vi "CRYReplace Statistics Curve Name.vi"(6 "IsMessage":bool, 8 "Hardware Setup In":string, 9 "Step Set up In":string, 10 "Setup in":T1={"No.VI"=0, "Category"="", "StepName"="", "Seq setup flattened"="", "Comment"="", "Steps config."=[], "Jump config"=[], "Start"=0.0, "Increment"=0.0, "Name"="Pa", "Unit"="Pa", "Y data"=1, "Y prefix"="", "Y dB ref"=1.0, "Y unit"="", "Repeat State Array"=[]} {"Repeat State Array"."Start" format="%#_5g"; "Y dB ref" format="%.1f"; "Y data" items=["dB", "Lin"]; "Start" format="%#_5g"}, 11 "Type In":string) -> (0 "RunFlag":bool, 3 "Inserted Names Out":string[](array[string]))   [LabVIEW 2013]
uses:
  Typedef Control/CRYStep.ctl
  Typedef Control/CRYData Cluster Array.ctl
  Typedef Control/CRYData Cluster.ctl
  CRYMainGlobal.vi
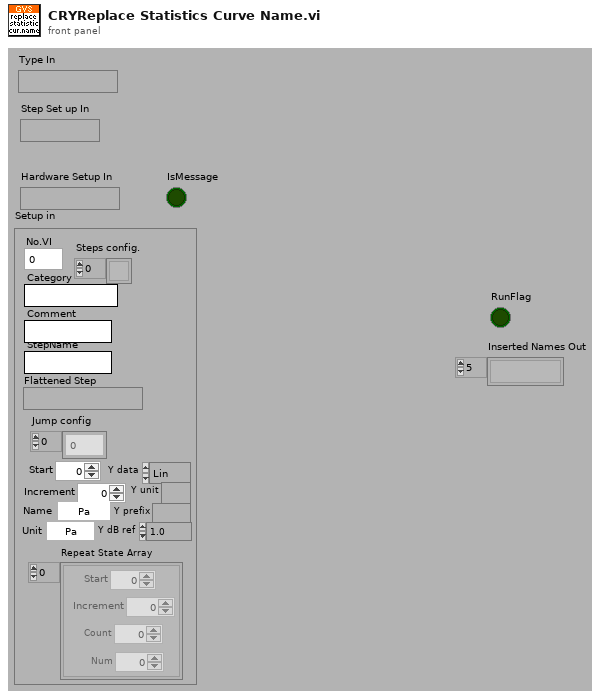
[diagram p1: front panel]
types:
  T1 = typedef "CRYStep.ctl" = cluster{"No.VI":i32, "Category":string, "StepName":string, "Seq setup flattened":string, "Comment":string, "Steps config.":bool[], "Jump config":i32[], "Start":dbl, "Increment":dbl, "Name":string, "Unit":string, "Y data":u16, "Y prefix":string, "Y dB ref":dbl, "Y unit":string, "Repeat State Array":cluster{"Start":dbl, "Increment":dbl, "Count":i32, "Num":i32}[]}
  T2 = typedef "CRYData Cluster Array.ctl" = T3[]
  T3 = typedef "CRYData Cluster.ctl" = cluster{"Name":string, "Curve":cluster{"x":dbl, "y":dbl, "z":dbl}[], "X data":u16, "Y data":u16, "Z data":u16, "X axis":u16, "Y axis":u16, "Z axis":u16, "X unit":string, "Y unit":string, "Z unit":string, "X dB ref":dbl, "Y dB ref":dbl, "Z dB ref":dbl, "single val":bool, "protected":bool, "display X":bool, "display Y":bool, "display Z":bool, "Test Info":string, "Step No.":i32, "Plot Settings":cluster{"Color":u32, "Interpolation":u8, "Point Style":u8, "Line Style":u8, "Point Color":u32, "Line Width":u8, "Bar Plot Style":u8, "Fill To":i16}, "AutoProtect":bool}
  T4 = cluster{"Start":dbl, "Increment":dbl, "Count":i32, "Num":i32}[]
  T5 = typedef "CRYStatistic cluster.ctl" = cluster{"Mode":u16, "No.Ranked(BF)":i32, "No.Ranked(WF)":i32, "Absolute Margin Standard Deviation":bool, "+/- sigma Res":i32, "Margin Standard Deviation":bool, "Margin Mean":bool, "Overall Yield":bool, "Individual Limits Yield":bool, "LSL Unit":string, "USL Unit\n":string, "LSL":dbl, "USL":dbl, "Worst Fit to Average":bool, "Best Fit to Average":bool, "Ppk":bool, "Pp":bool, "Absolute Standard Deviation":bool, "+/- sigma Dat":i32, "Standard Deviation ":bool, "Mean":bool, "Min ":bool, "Max ":bool, "No.of Curves Selected":i32, "Curves":string[], " Results":string[], "Name":string, "Help":string, "Tab Value":enum32{"Setting", "Help"}, "Work in":u16, "Mode xyz":u16}
  T6 = cluster{"Max ":bool, "Min ":bool, "Mean":bool, "Absolute Standard Deviation":bool, "Standard Deviation ":bool, "Pp":bool, "Ppk":bool, "Best Fit to Average":bool, "Worst Fit to Average":bool}
  T7 = cluster{"Individual Limits Yield":bool, "Overall Yield":bool, "Margin Mean":bool, "Absolute Margin Standard Deviation":bool, "Margin Standard Deviation":bool}
  T8 = typedef "CRYResult Cluster.ctl" = cluster{"Name":string, "Margin":dbl, "unit":string, "Verdict":bool, "Limit":string, "Max/Min":string, "protected":bool, "Step No.":i32, "Test Info":string, "AutoProtect":bool}
  T9 = enum32{"English", "Chinese", "Korean", "Japanese", "Russian", "Chinese traditional"}
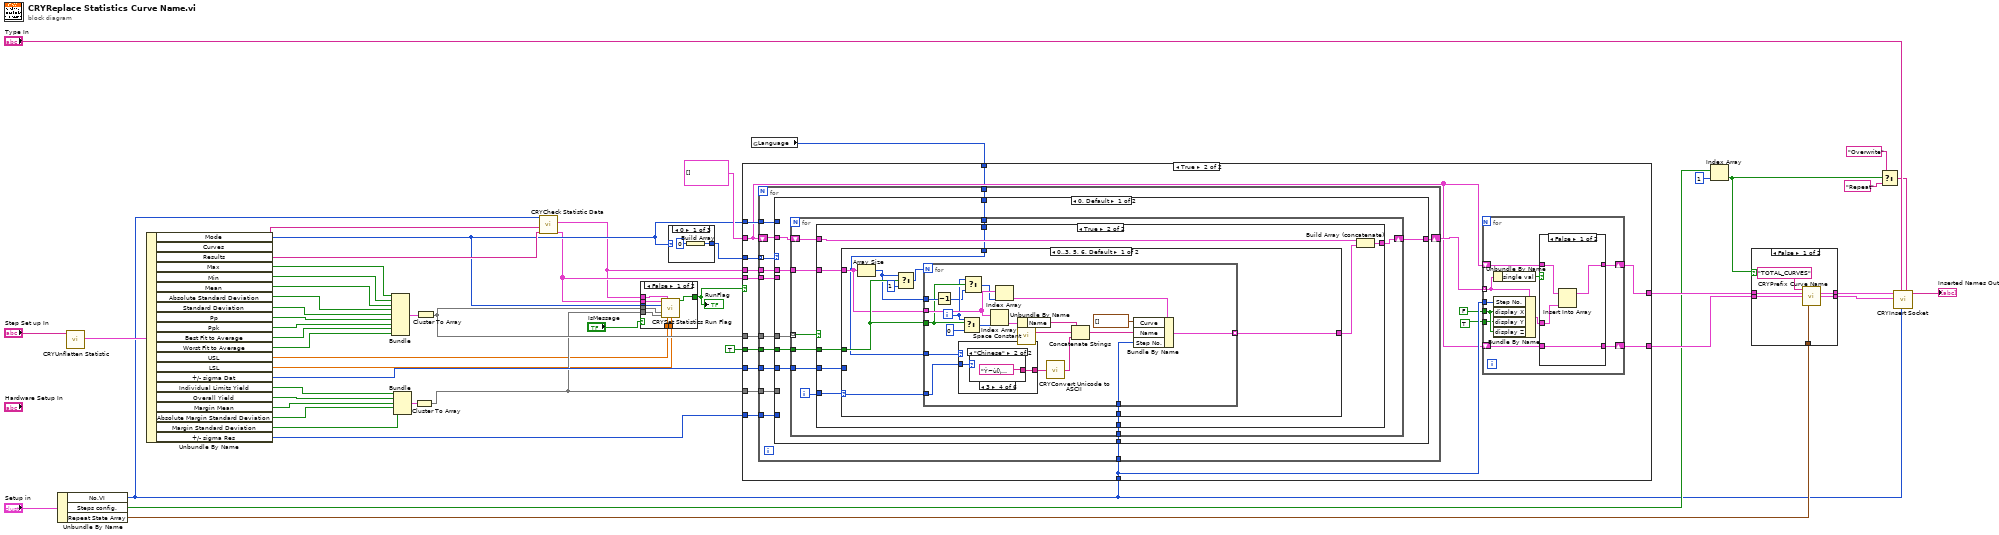
[diagram p0: block diagram]
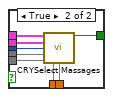
[diagram p2: hidden frame]
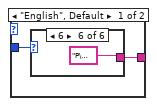
[diagram p6: hidden frame]
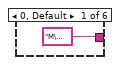
[diagram p7: hidden frame]
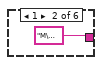
[diagram p8: hidden frame]
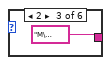
[diagram p9: hidden frame]
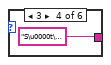
[diagram p10: hidden frame]
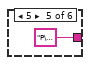
[diagram p11: hidden frame]
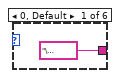
[diagram p12: hidden frame]
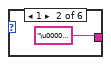
[diagram p13: hidden frame]
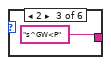
[diagram p14: hidden frame]
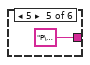
[diagram p15: hidden frame]
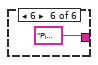
[diagram p16: hidden frame]
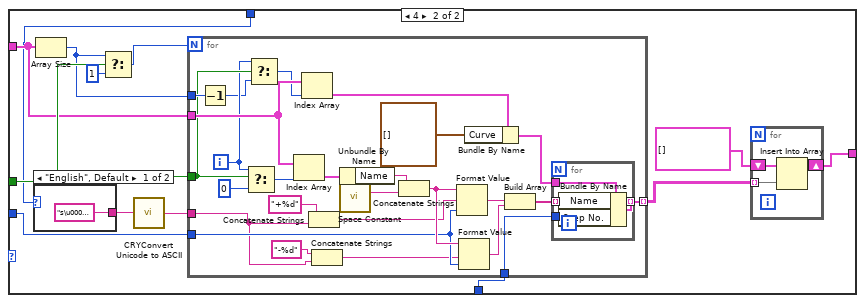
[diagram p17: hidden frame]
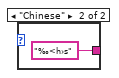
[diagram p18: hidden frame]
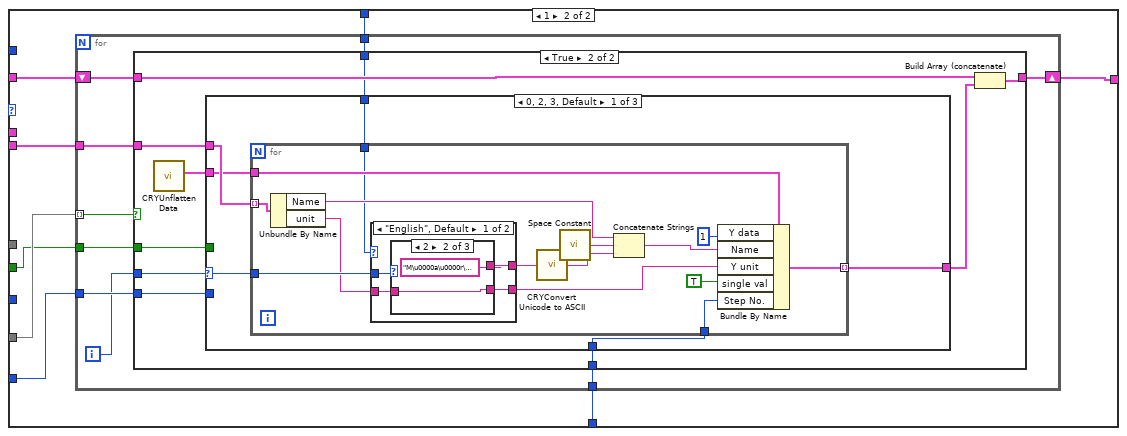
[diagram p19: hidden frame]
diagram:
  n1 = Unbundle By Name("Setup in") -> ("No.VI"=w10:i32, "Steps config."=w16:bool[], "Repeat State Array"=w15:T4)
  n2 = call "CRYUnflatten Statistic.vi"("Flatten Statistics"="Step Set up In") -> ("Statistics"=w29:T5)  [unwired: 10 out]
  n3 = Unbundle By Name(w29) -> ("Mode"=w9:u16, "Curves"=w12:string[], "Results"=w11:string[], "Max"=w47:bool, "Min"=w46:bool, "Mean"=w45:bool, "Absolute Standard Deviation"=w44:bool, "Standard Deviation"=w43:bool, "Pp"=w42:bool, "Ppk"=w41:bool, "Best Fit to Average"=w40:bool, "Worst Fit to Average"=w39:bool, "USL"=w6:dbl, "LSL"=w5:dbl, "+/- sigma Dat"=w32:i32, "Individual Limits Yield"=w37:bool, "Overall Yield"=w36:bool, "Margin Mean"=w35:bool, "Absolute Margin Standard Deviation"=w34:bool, "Margin Standard Deviation"=w33:bool, "+/- sigma Res"=w31:i32)
  n4 = Bundle("Max"=w47, "Min"=w46, "Mean"=w45, "Absolute Standard Deviation"=w44, "Standard Deviation"=w43, "Pp"=w42, "Ppk"=w41, "Best Fit to Average"=w40, "Worst Fit to Average"=w39) -> (w48:T6)  [unwired: 1 out]
  n5 = Bundle("Individual Limits Yield"=w37, "Overall Yield"=w36, "Margin Mean"=w35, "Absolute Margin Standard Deviation"=w34, "Margin Standard Deviation"=w33) -> (w38:T7)  [unwired: 1 out]
  n6 = Cluster To Array(cluster=w38) -> (array=w7:bool[])
  n7 = Cluster To Array(cluster=w48) -> (array=w8:bool[])
  n8 = call "CRYCheck Statistic Data.vi"("Results"=w11, "Curves"=w12, "No.VI"=w10) -> ("Result Out"=w4:T8[], "Data Out"=w3:T2)  [unwired: 7 in]
  n9 = case shown="False" "IsMessage" {
    tunnel: w9 -> [w56 w66]
    tunnel: w8 -> [w55 w65]
    tunnel: w7 -> [w54 w64]
    tunnel: w6 -> [w53 w63]
    tunnel: w5 -> [w52 w62]
    tunnel: w4 -> [w57 w61]
    tunnel: w3 -> [w58 w60]
    tunnel: [w51 w59] -> w2
    frame False {
      n10 = call "CRYSet Statistics Run Flag.vi"("Results in"=w57, "Data in"=w58, "Mode"=w56, "Dat_State"=w55, "Res_state"=w54, "USL"=w53, "LSL"=w52) -> ("Run flag"=w51:bool)  [unwired: 7 in, 1 out]
    }
    frame True {
      n11 = call "CRYSelect Massages.vi"("Data in"=w60, "Results in"=w61, "Mode"=w66, "Dat_State"=w65, "Res_state"=w64, "USL"=w63, "LSL"=w62) -> ("Run flag"=w59:bool)  [unwired: 3 in, 5 out]
    }
  }
  "RunFlag" <- w2
  n12 = case shown="0" w9 {
    tunnel: [w67 w69 w71] -> w30
    frame 0 {
      n13 = Build Array(0 ("No.Ranked(WF)")) -> (w67:i32[])
    }
    frame 1 {
      n14 = Build Array(1 ("No.Ranked(WF)")) -> (w69:i32[])
    }
    frame 2, Default {
      n15 = Build Array(0 ("No.Ranked(WF)"), 1 ("No.Ranked(WF)")) -> (w71:i32[])
    }
  }
  n16 = global read "CRYMainGlobal.vi" "Language"() -> (w13:T9)
  n17 = case shown="True" w2 {
    tunnel: w32 -> [_ w91]
    tunnel: w31 -> [_ w90]
    tunnel: w30 -> [_ w89]
    tunnel: w8 -> [_ w88]
    tunnel: w7 -> [_ w87]
    tunnel: w9 -> [_ w86]
    tunnel: TRUE ("On/Off Line") -> [_ w85]
    tunnel: w3 -> [_ w84]
    tunnel: w4 -> [_ w83]
    tunnel: [w74 w81] -> w22
    tunnel: [w74 w80] -> w21
    tunnel: w10 -> [_ w79]
    tunnel: T2 [] ("Data in") -> [w74 w78]
    tunnel: w13 -> [_ w77]
    frame False {
    }
    frame True {
      n18 = for {
        tunnel: w89 -> [w104] mode=indexing
        tunnel: w88 -> [w103]
        tunnel: w87 -> [w102]
        tunnel: w91 -> [w101]
        tunnel: w90 -> [w100]
        tunnel: w84 -> [w99]
        tunnel: w86 -> [w97]
        shift-right: [w96] -> w82
        shift-left: w78 -> [w98]
        tunnel: w85 -> [w95]
        tunnel: w83 -> [w94]
        tunnel: w79 -> [w93]
        tunnel: w77 -> [w92]
        n19 = case shown="0, Default" w104 {
          tunnel: w103 -> [w112 _]
          tunnel: w102 -> [_ w231]
          tunnel: w101 -> [w111 _]
          tunnel: w100 -> [_ w232]
          tunnel: w99 -> [w110 _]
          tunnel: w98 -> [w109 w230]
          tunnel: w97 -> [_ _]
          tunnel: [w108 w229] -> w96
          tunnel: w95 -> [w107 w227]
          tunnel: w94 -> [_ w228]
          tunnel: w93 -> [w106 w226]
          tunnel: w92 -> [w105 w225]
          frame 0, Default {
            n20 = for {
              tunnel: w112 -> [w120] mode=indexing
              tunnel: w111 -> [w121]
              tunnel: w110 -> [w118]
              shift-right: [w116] -> w108
              shift-left: w109 -> [w117]
              tunnel: w107 -> [w115]
              tunnel: w106 -> [w114]
              tunnel: w105 -> [w113]
              i -> [w119]
              n21 = case shown="True" w120 {
                tunnel: w119 -> [_ w129]
                tunnel: w121 -> [_ w125]
                tunnel: w118 -> [_ w128]
                tunnel: w117 -> [w122 w131]
                tunnel: [w122 w130] -> w116
                tunnel: w115 -> [_ w127]
                tunnel: w114 -> [_ w124]
                tunnel: w113 -> [_ w123]
                frame False {
                }
                frame True {
                  n22 = case shown="0..3, 5, 6, Default" w129 {
                    selector: w129 -> [w134 _]
                    tunnel: w128 -> [w137 w186]
                    tunnel: w127 -> [w138 w187]
                    tunnel: [w135 w181] -> w126
                    tunnel: w125 -> [_ w184]
                    tunnel: w124 -> [w133 w180]
                    tunnel: w123 -> [w132 w179]
                    frame 0..3, 5, 6, Default {
                      n23 = Array Size(array=w137) -> (size(s)=w136:i32)
                      n24 = Select(t=w136, s=w138, f=1) -> (s? t:f=w139:i32)
                      n25 = for {
                        N: w139 -> [_]
                        tunnel: w138 -> [w149]
                        tunnel: w137 -> [w156]
                        tunnel: w136 -> [w158]
                        tunnel: [w150] -> w135 mode=indexing
                        tunnel: w134 -> [w145]
                        tunnel: w133 -> [w144]
                        tunnel: w132 -> [w143]
                        i -> [w148]
                        n26 = Decrement(x=w158) -> (x-1=w147:i32)
                        n27 = case shown="\"Chinese\"" w143 {
                          tunnel: w145 -> [w162 w170]
                          tunnel: [w161 w169] -> w142
                          frame "English", Default {
                            n28 = case shown="6" w162 {
                              tunnel: ["M\u0000a\u0000x\u0000" ("string") "M\u0000i\u0000n\u0000" ("string") "M\u0000e\u0000a\u0000n\u0000" ("string") "S\u0000t\u0000d\u0000 \u0000D\u0000e\u0000v\u0000" ("string") "P\u0000p\u0000" ("string") "P\u0000p\u0000k\u0000" ("string")] -> w161
                              frame 0, Default {
                              }
                              frame 1 {
                              }
                              frame 2 {
                              }
                              frame 3 {
                              }
                              frame 5 {
                              }
                              frame 6 {
                              }
                            }
                          }
                          frame "Chinese" {
                            n29 = case shown="3" w170 {
                              tunnel: ["\u0000g'Y<P" ("string") "\u0000g\u000f\\<P" ("string") "s^GW<P" ("string") "Ý~ù[\u0007hÆQî]" ("string") "P\u0000p\u0000" ("string") "P\u0000p\u0000k\u0000" ("string")] -> w169
                              frame 0, Default {
                              }
                              frame 1 {
                              }
                              frame 2 {
                              }
                              frame 3 {
                              }
                              frame 5 {
                              }
                              frame 6 {
                              }
                            }
                          }
                        }
                        n30 = Select(t=w148, s=w149, f=0) -> (s? t:f=w159:i32)
                        n31 = Select(t=w148, s=w149, f=w147) -> (s? t:f=w146:i32)
                        n32 = Index Array(array=w156, index=w159) -> (element=w157:T3)
                        n33 = Index Array(array=w156, index=w146) -> (element=w153:T3)
                        n34 = Unbundle By Name(w157) -> ("Name"=w155:string)
                        n35 = call <vilib>:"Space Constant.vi"() -> ("String"=w154:string)
                        n36 = call "CRYConvert Unicode to ASCII.vi"("Unicode"=w142) -> ("ASCII"=w141:string)  [unwired: 4 in]
                        n37 = Concatenate Strings(w155, w154, w141) -> (w152:string)
                        n38 = Bundle By Name(cluster=w153, "Curve"=cluster{"x":dbl, "y":dbl, "z":dbl}[] [], "Name"=w152, "Step No."=w144) -> (w150:T3)
                      }
                    }
                    frame 4 {
                      n39 = case shown="\"English\", Default" w179 {
                        tunnel: ["s\u0000i\u0000g\u0000m\u0000a\u0000" ("format string") "‰<h›s" ("format string")] -> w178
                        frame "English", Default {
                        }
                        frame "Chinese" {
                        }
                      }
                      n40 = Array Size(array=w186) -> (size(s)=w185:i32)
                      n41 = Select(t=w185, s=w187, f=1) -> (s? t:f=w188:i32)
                      n42 = call "CRYConvert Unicode to ASCII.vi"("Unicode"=w178) -> ("ASCII"=w177:string)  [unwired: 4 in]
                      n43 = for {
                        N: w188 -> [_]
                        tunnel: w187 -> [w211]
                        tunnel: w186 -> [w216]
                        tunnel: w185 -> [w218]
                        tunnel: w184 -> [w200]
                        tunnel: [w202] -> w182 mode=indexing
                        tunnel: w180 -> [w201]
                        tunnel: w177 -> [w197]
                        i -> [w210]
                        n44 = Decrement(x=w218) -> (x-1=w209:i32)
                        n45 = Select(t=w210, s=w211, f=0) -> (s? t:f=w219:i32)
                        n46 = Select(t=w210, s=w211, f=w209) -> (s? t:f=w208:i32)
                        n47 = Index Array(array=w216, index=w219) -> (element=w217:T3)
                        n48 = Index Array(array=w216, index=w208) -> (element=w213:T3)
                        n49 = Concatenate Strings("+%d" ("format string"), w197) -> (w196:string)
                        n50 = Concatenate Strings("-%d" ("format string"), w197) -> (w195:string)
                        n51 = Unbundle By Name(w217) -> ("Name"=w215:string)
                        n52 = call <vilib>:"Space Constant.vi"() -> ("String"=w214:string)
                        n53 = Concatenate Strings(w215, w214) -> (w205:string)
                        n54 = Format Value(string ("")=w205, format string=w196, value (0)=w200) -> (output string=w206:string)
                        n55 = Format Value(string ("")=w205, format string=w195, value (0)=w200) -> (output string=w207:string)
                        n56 = Bundle By Name(cluster=w213, "Curve"=cluster{"x":dbl, "y":dbl, "z":dbl}[] []) -> (w203:T3)
                        n57 = Build Array(w206, w207) -> (w204:string[])
                        n58 = for {
                          tunnel: w204 -> [w224] mode=indexing
                          tunnel: w203 -> [w223]
                          tunnel: [w222] -> w202 mode=indexing
                          tunnel: w201 -> [w221]
                          n59 = Bundle By Name(cluster=w223, "Name"=w224, "Step No."=w221) -> (w222:T3)
                        }
                      }
                      n60 = for {
                        tunnel: w182 -> [w194] mode=indexing
                        shift-right: [w192] -> w181
                        shift-left: T2 [] ("Data in") -> [w193]
                        n61 = Insert Into Array(array=w193, new element=w194) -> (w192:T2)  [unwired: 1 in]
                      }
                    }
                  }
                  n62 = Build Array (concatenate)(w131, w126) -> (w130:T2)
                }
              }
            }
          }
          frame 1 {
            n63 = for {
              tunnel: w231 -> [w241] mode=indexing
              tunnel: w232 -> [w240]
              shift-right: [w237] -> w229
              shift-left: w230 -> [w238]
              tunnel: w228 -> [w236]
              tunnel: w227 -> [w235]
              tunnel: w226 -> [w234]
              tunnel: w225 -> [w233]
              i -> [w239]
              n64 = case shown="True" w241 {
                tunnel: w239 -> [_ w250]
                tunnel: w240 -> [_ w245]
                tunnel: w238 -> [w242 w252]
                tunnel: [w242 w251] -> w237
                tunnel: w236 -> [_ w249]
                tunnel: w235 -> [_ w246]
                tunnel: w234 -> [_ w244]
                tunnel: w233 -> [_ w243]
                frame False {
                }
                frame True {
                  n65 = call "CRYUnflatten Data.vi"() -> ("Datum"=w248:T3)  [unwired: 9 in, 2 out]
                  n66 = case shown="0, 2, 3, Default" w250 {
                    selector: w250 -> [w255 _ _]
                    tunnel: w249 -> [w258 w302 w319]
                    tunnel: w248 -> [w257 w307 w318]
                    tunnel: [w256 w298 w314] -> w247
                    tunnel: w246 -> [_ w303 _]
                    tunnel: w245 -> [_ _ w317]
                    tunnel: w244 -> [w254 w297 w313]
                    tunnel: w243 -> [w253 w294 w311]
                    frame 0, 2, 3, Default {
                      n67 = for {
                        tunnel: w258 -> [w271] mode=indexing
                        tunnel: w257 -> [w267]
                        tunnel: [w266] -> w256 mode=indexing
                        tunnel: w255 -> [w264]
                        tunnel: w254 -> [w262]
                        tunnel: w253 -> [w261]
                        n68 = Unbundle By Name(w271) -> ("Name"=w272:string, "unit"=w263:string)
                        n69 = case shown="\"English\", Default" w261 {
                          tunnel: [w277 w287] -> w260
                          tunnel: [w276 w286] -> w270
                          tunnel: w264 -> [w275 w285]
                          tunnel: w263 -> [w274 w284]
                          frame "English", Default {
                            n70 = case shown="2" w275 {
                              tunnel: ["Y\u0000i\u0000e\u0000l\u0000d\u0000" "M\u0000a\u0000r\u0000g\u0000i\u0000n\u0000 \u0000M\u0000e\u0000a\u0000n\u0000" ("string") "S\u0000t\u0000d\u0000 \u0000D\u0000e\u0000v\u0000" ("string")] -> w277
                              tunnel: ["%\u0000" ("Y unit") w280 w282] -> w276
                              tunnel: w274 -> [_ w280 w282]
                              frame 0, Default {
                              }
                              frame 2 {
                              }
                              frame 3 {
                              }
                            }
                          }
                          frame "Chinese" {
                            n71 = case shown="3" w285 {
                              tunnel: ["\bT<h" ("Unicode") ":Sô•s^GW<P" ("string") "\u0007hÆQî]" ("string")] -> w287
                              tunnel: ["%\u0000" ("Y unit") w290 w292] -> w286
                              tunnel: w284 -> [_ w290 w292]
                              frame 0, Default {
                              }
                              frame 2 {
                              }
                              frame 3 {
                              }
                            }
                          }
                        }
                        n72 = call "CRYConvert Unicode to ASCII.vi"("Unicode"=w260) -> ("ASCII"=w259:string)  [unwired: 4 in]
                        n73 = call <vilib>:"Space Constant.vi"() -> ("String"=w273:string)
                        n74 = Concatenate Strings(w272, w273, w259) -> (w268:string)
                        n75 = Bundle By Name(cluster=w267, "Y data"=u16 1, "Name"=w268, "Y unit"=w270, "single val"=TRUE, "Step No."=w262) -> (w266:T3)
                      }
                    }
                    frame 1 {
                      n76 = Index Array(array=w302) -> (element=w301:T8)  [unwired: 1 in]
                      n77 = Unbundle By Name(w301) -> ("Name"=w300:string)
                      n78 = case shown="\"English\", Default" w294 {
                        tunnel: w303 -> [_ _]
                        tunnel: w300 -> [_ _]
                        tunnel: ["O\u0000v\u0000e\u0000r\u0000a\u0000l\u0000l\u0000 \u0000Y\u0000i\u0000e\u0000l\u0000d\u0000" ";`\bT<h"] -> w296
                        frame "English", Default {
                        }
                        frame "Chinese" {
                        }
                      }
                      n79 = call "CRYConvert Unicode to ASCII.vi"("Unicode"=w296) -> ("ASCII"=w295:string)  [unwired: 4 in]
                      n80 = Bundle By Name(cluster=w307, "Y data"=u16 1, "Name"=w295, "Y unit"="%", "single val"=TRUE, "Step No."=w297) -> (w299:T3)
                      n81 = Build Array(w299) -> (w298:T3[])
                    }
                    frame 4 {
                      n82 = case shown="\"Chinese\"" w311 {
                        tunnel: ["s\u0000i\u0000g\u0000m\u0000a\u0000" "‰<h›s"] -> w310
                        frame "English", Default {
                        }
                        frame "Chinese" {
                        }
                      }
                      n83 = call "CRYConvert Unicode to ASCII.vi"("Unicode"=w310) -> ("ASCII"=w312:string)  [unwired: 4 in]
                      n84 = for {
                        tunnel: w319 -> [w342] mode=indexing
                        tunnel: w318 -> [w340]
                        tunnel: w317 -> [w335]
                        tunnel: [w332] -> w315 mode=indexing
                        tunnel: w313 -> [w331]
                        tunnel: w312 -> [w326]
                        n85 = Unbundle By Name(w342) -> ("unit"=w338:string, "Name"=w330:string)
                        n86 = Concatenate Strings("-%d", w326) -> (w327:string)
                        n87 = Concatenate Strings("+%d", w326) -> (w329:string)
                        n88 = Format Value(string ("")=w330, format string=w327, value (0)=w335) -> (output string=w337:string)
                        n89 = Format Value(string ("")=w330, format string=w329, value (0)=w335) -> (output string=w336:string)
                        n90 = Build Array(w336, w337) -> (w334:string[])
                        n91 = Bundle By Name(cluster=w340, "Y data"=u16 1, "Y unit"=w338, "single val"=TRUE) -> (w333:T3)
                        n92 = for {
                          tunnel: w334 -> [w346] mode=indexing
                          tunnel: w333 -> [w345]
                          tunnel: [w344] -> w332 mode=indexing
                          tunnel: w331 -> [w343]
                          n93 = Bundle By Name(cluster=w345, "Name"=w346, "Step No."=w343) -> (w344:T3)
                        }
                      }
                      n94 = for {
                        tunnel: w315 -> [w324] mode=indexing
                        shift-right: [w322] -> w314
                        shift-left: T2 [] ("Data in") -> [w323]
                        n95 = Insert Into Array(array=w323, new element=w324) -> (w322:T2)  [unwired: 1 in]
                      }
                    }
                  }
                  n96 = Build Array (concatenate)(w252, w247) -> (w251:T2)
                }
              }
            }
          }
        }
      }
      n97 = for {
        tunnel: w82 -> [w351] mode=indexing
        shift-right: [w354] -> w80
        shift-left: w78 -> [w355]
        shift-right: [w352] -> w81
        shift-left: w78 -> [w353]
        tunnel: w79 -> [w350]
        tunnel: FALSE -> [w348]
        tunnel: TRUE -> [w347]
        n98 = Unbundle By Name(w351) -> ("single val"=w356:bool)
        n99 = Bundle By Name(cluster=w351, "Step No."=w350, "display X"=w348, "display Y"=w347, "display Z"=w348) -> (w349:T3)
        n100 = case shown="False" w356 {
          tunnel: w349 -> [w357 w361]
          tunnel: w355 -> [w358 w364]
          tunnel: [w358 w363] -> w354
          tunnel: w353 -> [w360 w362]
          tunnel: [w359 w362] -> w352
          frame False {
            n101 = Insert Into Array(array=w360, new element=w357) -> (w359:T2)  [unwired: 1 in]
          }
          frame True {
            n102 = Insert Into Array(array=w364, new element=w361) -> (w363:T2)  [unwired: 1 in]
          }
        }
      }
    }
  }
  n103 = Index Array(array=w16, index=1) -> (element=w18:bool)
  n104 = case shown="False" w18 {
    tunnel: w22 -> [w369 w372]
    tunnel: w21 -> [w368 w371]
    tunnel: [w367 w372] -> w20
    tunnel: [w366 w371] -> w19
    tunnel: w15 -> [w365 _]
    frame False {
      n105 = call "CRYPrefix Curve Name.vi"("Type In"="TOTAL_CURVES", "Curves In"=w369, "Values In"=w368, "Repeat State Array In"=w365) -> ("Curves Out"=w367:T2, "Values Out"=w366:T2)  [unwired: 8 in, 2 out]
    }
    frame True {
    }
  }
  n106 = Select(t="Overwrite" ("Y unit"), s=w18, f="Repeat") -> (s? t:f=w23:string)
  n107 = call "CRYInsert Socket.vi"("sOption2"=w23, "Step No."=w10, "sOption1"="Type In", "Values"=w19, "Curves"=w20) -> ("Inserted Names Out"=→"Inserted Names Out":string[])  [unwired: 6 in]
